vi "Sequence - Check Test Equipment.vi"(8 "error in (no error)":errorcluster) -> (0 "error out":errorcluster, 3 "PASS":bool)   [LabVIEW 2020]
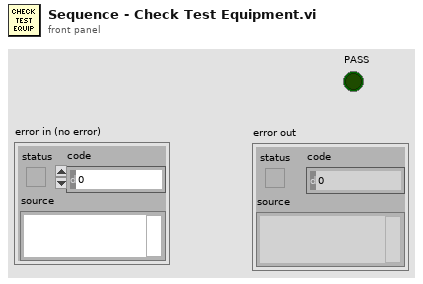
[diagram p1: front panel]
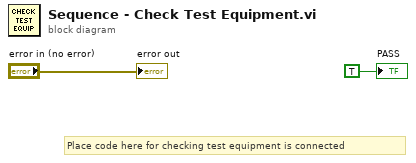
[diagram p0: block diagram]
diagram:
  # "Place code here for checking test equipment is connected"
  "error out" <- "error in (no error)"
  "PASS" <- TRUE ("PASS")
